vi "Wrapper.vi"(0 "IVI Refnum in":refnum<k15>="Dev1" caption="Load DMM", 1 "Current Level":dbl, 2 "Load SMU Channel":string, 3 "Load SMU":T1 {"Resolution in Digits" items=["3 1/2"=3.5, "4 1/2"=4.5, "5 1/2"=5.5, "6 1/2"=6.5, "7 1/2"=7.5]; "Range (Amps)" format="%.2p"}, 5 "Load SMU 2":refnum<k15>, 7 "Current Level Range":dbl, 9 "Voltage Limit":dbl, 11 "error in (no error)":errorcluster, 12 "Voltage Limit Range":dbl, 13 "Source Delay (Sec)":dbl) -> (4 "Numeric 2":dbl, 6 "Numeric":dbl, 8 "Name":T2, 10 "Measurement":dbl, 14 "Over Range?":bool, 15 "error out":errorcluster)   [LabVIEW 2021, in "Test Case T12.lvlib"]
uses:
  Test Case T12.lvlib
  NIDMM/Meas T12.ctl
  NIDMM/LoadDMM t12.ctl
  NIDCpower/NIDCPower T12.lvlib
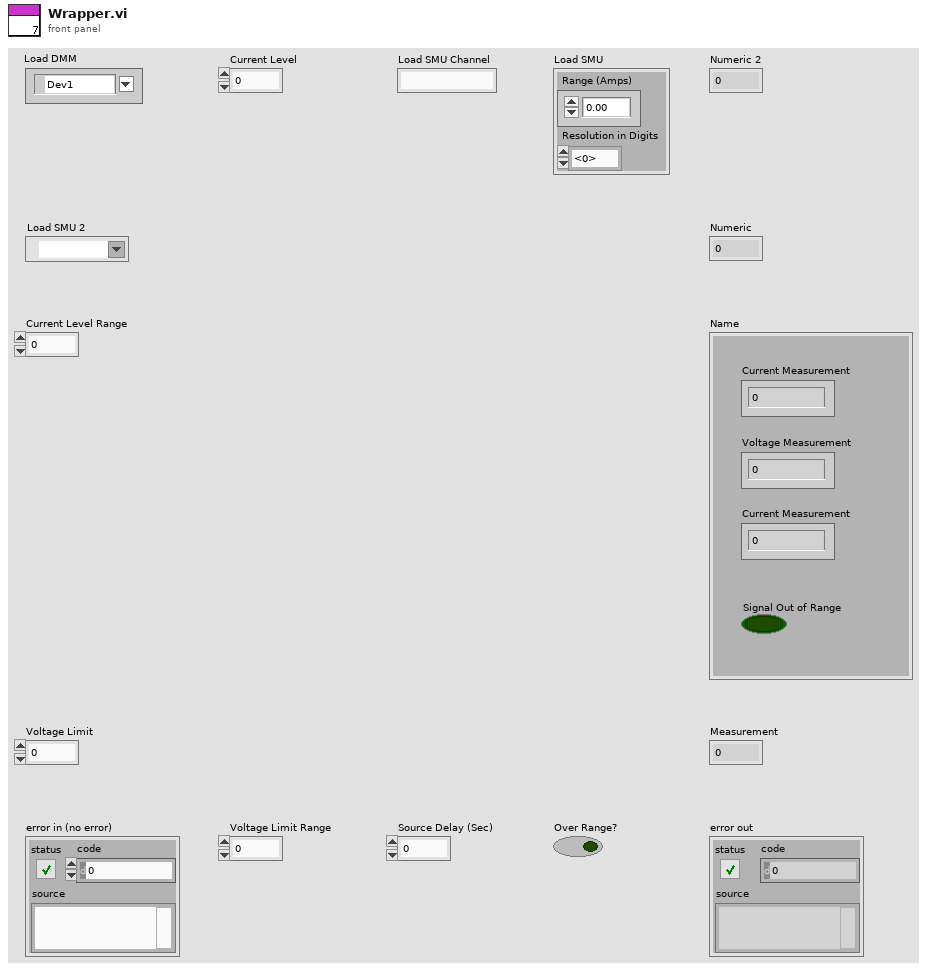
[diagram p1: front panel]
types:
  T1 = typedef "LoadDMM t12.ctl" = cluster{"Range (Amps)":dbl, "Resolution in Digits":dbl}
  T2 = typedef "Meas T12.ctl" = cluster{"Current Measurement":dbl, "Voltage Measurement":dbl, "Signal Out of Range":bool, "Current in DMM":dbl}
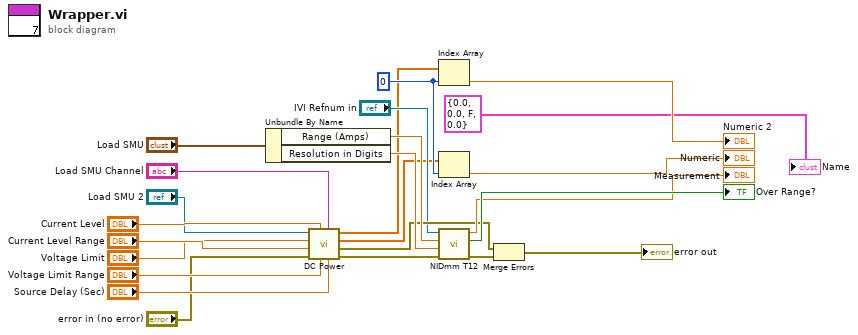
[diagram p0: block diagram]
diagram:
  w3 = 0 ("index")
  n1 = Unbundle By Name("Load SMU") -> ("Range (Amps)"=w18:dbl, "Resolution in Digits"=w19:dbl)
  n2 = call "DC Power.vi"("Source Delay (Sec)"="Source Delay (Sec)", "Load SMU Channel"="Load SMU Channel", "Voltage Limit Range"="Voltage Limit Range", "Current Level"="Current Level", "error in (no error)"="error in (no error)", "Current Level Range"="Current Level Range", "Voltage Limit"="Voltage Limit", "IVI Refnum in"="Load SMU 2") -> (0:"error out"=w9:errorcluster, 1:"error out"=w10:errorcluster, "current measurements"=w2:dbl[], "voltage measurements"=w1:dbl[])
  n3 = Index Array(array=w1, index=w3) -> (element=→"Numeric 2":dbl)
  n4 = Index Array(array=w2, index=w3) -> (element=→"Numeric":dbl)
  n5 = call "NIDmm T12.vi"("error in (no error)"=w9, "Range (Amps)"=w19, "Resolution in Digits"=w18, "IVI Refnum in"="IVI Refnum in") -> ("error out"=w11:errorcluster, "Over Range?"=→"Over Range?":bool, "Measurement"=→"Measurement":dbl)  [unwired: 5 in]
  n6 = Merge Errors(w10, w11) -> (→"error out":errorcluster)
  "Name" <- T2 {"Current Measurement"=0.0, "Voltage Measurement"=0.0, "Signal Out of Range"=FALSE, "Current in DMM"=0.0} ("Name")
